vi "FPGA_SuspensionCurrentCheck.vi"() -> ()   [LabVIEW 2014]
uses:
  <vilib>/rvi/Memory/Memory_Emulation/nirvimemoryFastEmulation.vi
  <vilib>/rvi/Memory/Memory_Emulation/nirvimemoryEmulation.vi
  <vilib>/rvi/Emulation/niFpgaEmulationIsFPGAContextNoSignature.vi
  <vilib>/rvi/DataTransferAndStorage/Container/Common/niFpgaContainerGetUniqueNameForEmu.vi
  <vilib>/rvi/Emulation/niFpgaProcessEmulError.vi
  <vilib>/rvi/Emulation/niFpgaSctlEmulationGetInTimedLoop.vi
  <vilib>/rvi/errors/nirviReportUnexpectedCaseInternalError (U32).vi
  <vilib>/rvi/eio/common/nirviEmuTemplateMethod_errors.vi
  <vilib>/rvi/interface/RandomDataEmulation/niFpgaRandomDataHandleErrors.vi
  <vilib>/rvi/Emulation/niFpgaGetClockAttributes.vi
  <vilib>/rvi/Emulation/niFpgaEmulationReportErrorSimple.vi
  <vilib>/rvi/Emulation/niFpgaCriticalErrorInLSC.vi
  <vilib>/rvi/DataTransferAndStorage/Container/XNode/niFpgaContainer.xnode
  <vilib>/eio/EIONode/EIONode.xnode
  <vilib>/rvi/interface/RandomDataEmulation/nirviRandomDataFpgaReadWriteTemplate.vi
panel:
  in  "StepPulseIndex":u32
  in  "SampleSleep us":i32
  in  "SampleNumPerStepIn":i32
  in  "StepInNum":i32
  in  "StepIn?":bool
  in  "SampleNumAfterBack":i32
  out "Monitor":i32
  out "PresCurrent":i16
  out "ZPos":i16
  out "Finished?":bool
  out "Arrived?":bool
  in  "sleep us":u32
  in  "stop":bool
  in  "threshold":sgl
  in  "Offset":i16
  in  "SampleNumAfterApproached":i32
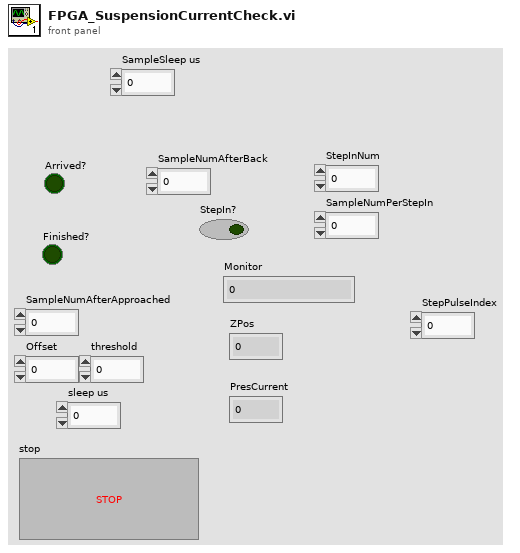
[diagram p1: front panel]
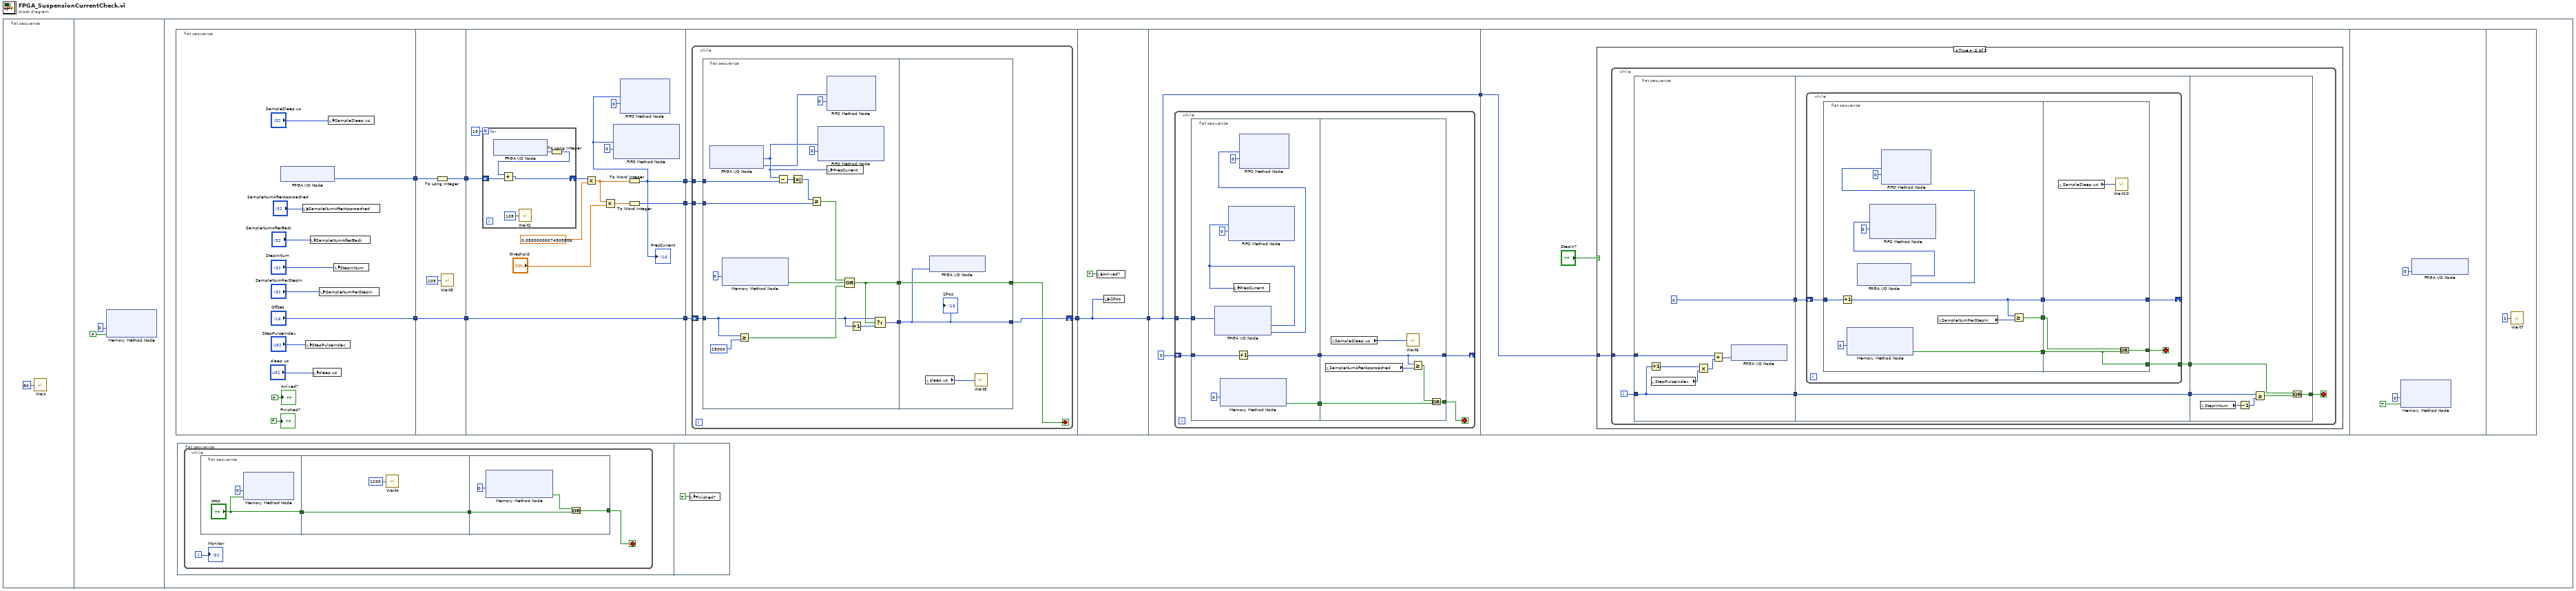
[diagram p0: block diagram]
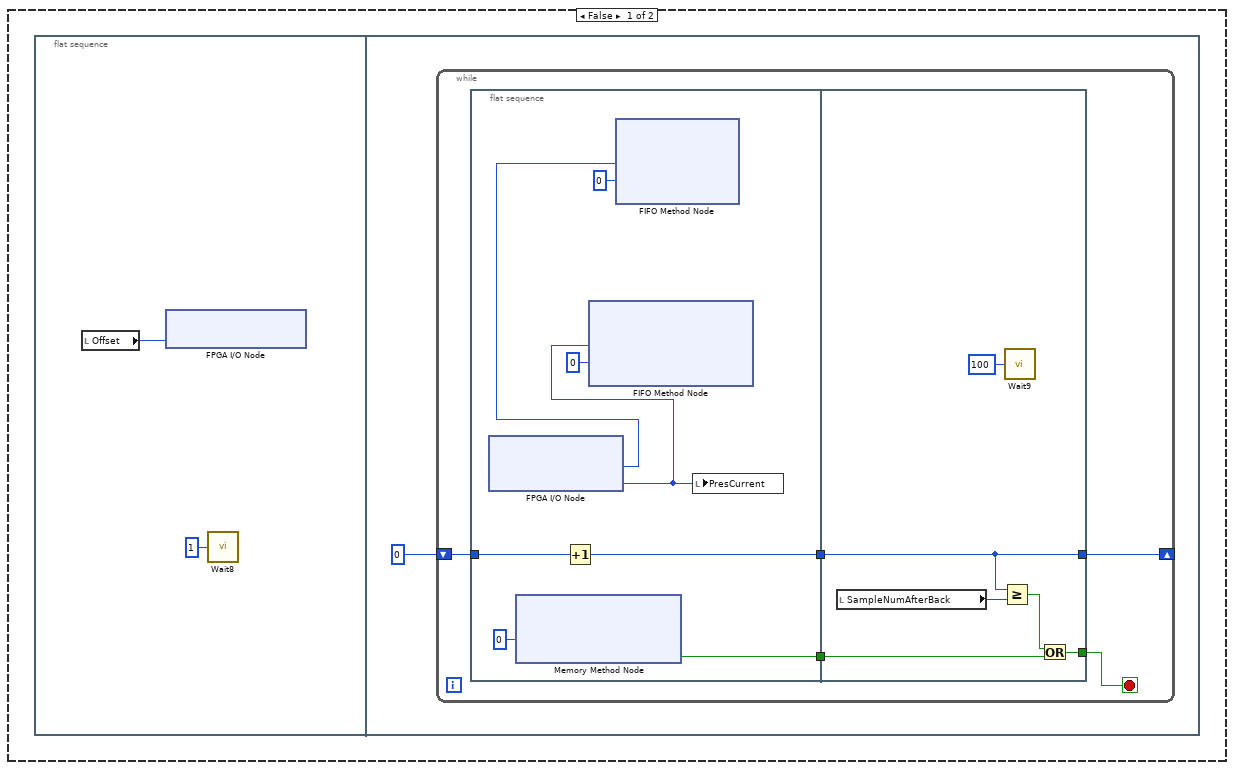
[diagram p2: hidden frame]
diagram:
  n1 = flat-sequence {
    frame #0 {
      n2 = call "Wait"("Count(mSec)"=u32 80) -> ()  [unwired: 1 out]
    }
    frame #1 {
      n3 = xnode ("Memory Method Node")("Address"=u32 0, "Data"=FALSE) -> ()  [unwired: 1 in, 1 out]
    }
    frame #2 {
      n4 = flat-sequence {
        tunnel: ["Offset"] -> w13
        tunnel: [w35] -> w12
        tunnel: w13 -> [w41]
        tunnel: [w41] -> w11
        tunnel: [w38] -> w10
        tunnel: w12 -> [w39]
        tunnel: w11 -> [w53]
        tunnel: [w53] -> w9
        tunnel: w10 -> [w51]
        tunnel: [w43] -> w8
        tunnel: [w45] -> w7
        tunnel: w9 -> [w62]
        tunnel: w8 -> [w61]
        tunnel: w7 -> [w60]
        tunnel: [w59] -> w6
        tunnel: w6 -> [w90]
        tunnel: [w90] -> w5
        tunnel: w5 -> [w92]
        tunnel: [w92] -> w4
        tunnel: w4 -> [w115]
        frame #0 {
          n5 = xnode "FPGA I/O Node"() -> ("Connector0/AI1"=w35:i16)  [unwired: 1 in, 1 out]
          n6 = local write "SampleNumAfterApproached"("SampleNumAfterApproached") -> ()
          n7 = local write "StepPulseIndex"("StepPulseIndex") -> ()
          n8 = local write "SampleNumAfterBack"("SampleNumAfterBack") -> ()
          n9 = local write "sleep us"("sleep us") -> ()
          n10 = local write "SampleNumPerStepIn"("SampleNumPerStepIn") -> ()
          n11 = local write "SampleSleep us"("SampleSleep us") -> ()
          n12 = local write "StepInNum"("StepInNum") -> ()
          "Arrived?" <- FALSE ("Arrived?")
          "Finished?" <- FALSE ("Arrived?")
        }
        frame #1 {
          n13 = To Long Integer(number=w39) -> (32bit integer=w38:i32)
          n14 = call "Wait3"("Count(uSec)"=u32 105) -> ()  [unwired: 1 out]
        }
        frame #2 {
          n15 = for {
            N: 19 -> [_]
            shift-right: [w54] -> w50
            shift-left: w51 -> [w57]
            n16 = xnode "FPGA I/O Node"() -> ("Connector0/AI1"=w56:i16)  [unwired: 1 in, 1 out]
            n17 = call "Wait2"("Count(uSec)"=u32 105) -> ()  [unwired: 1 out]
            n18 = To Long Integer(number=w56) -> (32bit integer=w55:i32)
            n19 = Add(x=w55, y=w57) -> (x+y=w54:i32)
          }
          n20 = Multiply(x=w50, y=sgl 0.05) -> (x*y=w47:sgl)
          n21 = Multiply(x=w47, y="threshold") -> (x*y=w46:sgl)
          n22 = To Word Integer(number=w47) -> (16bit integer=w43:i16)
          "PresCurrent" <- w43
          n23 = xnode ("FIFO Method Node")("Element"=w43, "Timeout"=0) -> ()  [unwired: 1 in, 2 out]
          n24 = xnode ("FIFO Method Node")("Element"=w43, "Timeout"=0) -> ()  [unwired: 1 in, 2 out]
          n25 = To Word Integer(number=w46) -> (16bit integer=w45:i16)
        }
        frame #3 {
          n26 = while {
            shift-right: [w65] -> w59
            shift-left: w62 -> [w67]
            tunnel: w61 -> [w69]
            tunnel: w60 -> [w68]
            stop <- w63 stop-if-true
            n27 = flat-sequence {
              tunnel: w69 -> [w86]
              tunnel: w68 -> [w84]
              tunnel: w67 -> [w76]
              tunnel: [w74] -> w66
              tunnel: [w73] -> w64
              tunnel: w66 -> [w89]
              tunnel: [w89] -> w65
              tunnel: [w87] -> w63
              tunnel: w64 -> [w87]
              frame #0 {
                n28 = xnode "FPGA I/O Node"() -> ("Connector0/AI1"=w72:i16, "Connector0/AI0"=w70:i16)  [unwired: 2 in, 2 out]
                n29 = xnode ("Memory Method Node")("Address"=u32 0) -> ("Data"=w78:bool)  [unwired: 1 in, 1 out]
                n30 = Greater Or Equal?(x=w76, y=i16 29000) -> (x >= y?=w77:bool)
                n31 = Subtract(x=w72, y=w86) -> (x-y=w85:i16)
                n32 = Absolute Value(x=w85) -> (abs(x)=w83:i16)
                n33 = Greater Or Equal?(x=w83, y=w84) -> (x >= y?=w79:bool)
                n34 = xnode ("FIFO Method Node")("Element"=w72, "Timeout"=0) -> ()  [unwired: 1 in, 2 out]
                n35 = xnode ("FIFO Method Node")("Element"=w70, "Timeout"=0) -> ()  [unwired: 1 in, 2 out]
                n36 = local write "PresCurrent"(w72) -> ()
                n37 = Compound Arithmetic op=OR(w79, w78, w77) -> (w73:bool)
                n38 = Increment(x=w76) -> (x+1=w75:i16)
                n39 = Select(t=w76, s=w73, f=w75) -> (s? t:f=w74:i16)
              }
              frame #1 {
                n40 = local read "sleep us"() -> (w88:u32)
                n41 = xnode "FPGA I/O Node"("Connector0/AO0"=w89) -> ()  [unwired: 1 in, 1 out]
                n42 = call "Wait5"("Count(uSec)"=w88) -> ()  [unwired: 1 out]
                "ZPos" <- w89
              }
            }
          }
        }
        frame #4 {
          n43 = local write "Arrived?"(TRUE ("Arrived?")) -> ()
          n44 = local write "ZPos"(w90) -> ()
        }
        frame #5 {
          n45 = while {
            tunnel: w92 -> [w99]
            shift-right: [w94] -> _
            shift-left: 0 -> [w96]
            stop <- w97 stop-if-true
            n46 = flat-sequence {
              tunnel: w99 -> [w108]
              tunnel: [w105] -> w98
              tunnel: w96 -> [w104]
              tunnel: [w103] -> w95
              tunnel: [w112] -> w97
              tunnel: w98 -> [w111]
              tunnel: w95 -> [w113]
              tunnel: [w113] -> w94
              frame #0 {
                n47 = xnode "FPGA I/O Node"("Connector0/AO0"=w108) -> ("Connector0/AI1"=w102:i16, "Connector0/AI0"=w100:i16)  [unwired: 3 in, 3 out]
                n48 = xnode ("Memory Method Node")("Address"=u32 0) -> ("Data"=w105:bool)  [unwired: 1 in, 1 out]
                n49 = xnode ("FIFO Method Node")("Element"=w102, "Timeout"=0) -> ()  [unwired: 1 in, 2 out]
                n50 = local write "PresCurrent"(w102) -> ()
                n51 = Increment(x=w104) -> (x+1=w103:i32)
                n52 = xnode ("FIFO Method Node")("Element"=w100, "Timeout"=0) -> ()  [unwired: 1 in, 2 out]
              }
              frame #1 {
                n53 = local read "SampleNumAfterApproached"() -> (w114:i32)
                n54 = local read "SampleSleep us"() -> (w109:i32)
                n55 = call "Wait6"("Count(uSec)"=w109) -> ()  [unwired: 1 out]
                n56 = Greater Or Equal?(x=w113, y=w114) -> (x >= y?=w110:bool)
                n57 = Or(x=w110, y=w111) -> (x .or. y?=w112:bool)
              }
            }
          }
        }
        frame #6 {
          n58 = case shown="True" "StepIn?" {
            tunnel: w115 -> [_ w139]
            frame False {
              n59 = flat-sequence {
                frame #0 {
                  n60 = local read "Offset"() -> (w118:i16)
                  n61 = xnode "FPGA I/O Node"("Connector0/AO0"=w118) -> ()  [unwired: 1 in, 1 out]
                  n62 = call "Wait8"("Count(mSec)"=u32 1 ("Count(uSec)")) -> ()  [unwired: 1 out]
                }
                frame #1 {
                  n63 = while {
                    shift-right: [w122] -> _
                    shift-left: 0 -> [w124]
                    stop <- w121 stop-if-true
                    n64 = flat-sequence {
                      tunnel: w124 -> [w132]
                      tunnel: [w131] -> w123
                      tunnel: [w129] -> w120
                      tunnel: w123 -> [w138]
                      tunnel: [w138] -> w122
                      tunnel: [w134] -> w121
                      tunnel: w120 -> [w136]
                      frame #0 {
                        n65 = xnode "FPGA I/O Node"() -> ("Connector0/AI0"=w127:i16, "Connector0/AI1"=w128:i16)  [unwired: 2 in, 2 out]
                        n66 = xnode ("Memory Method Node")("Address"=u32 0) -> ("Data"=w129:bool)  [unwired: 1 in, 1 out]
                        n67 = Increment(x=w132) -> (x+1=w131:i32)
                        n68 = xnode ("FIFO Method Node")("Element"=w128, "Timeout"=0) -> ()  [unwired: 1 in, 2 out]
                        n69 = xnode ("FIFO Method Node")("Element"=w127, "Timeout"=0) -> ()  [unwired: 1 in, 2 out]
                        n70 = local write "PresCurrent"(w128) -> ()
                      }
                      frame #1 {
                        n71 = local read "SampleNumAfterBack"() -> (w137:i32)
                        n72 = Greater Or Equal?(x=w138, y=w137) -> (x >= y?=w135:bool)
                        n73 = call "Wait9"("Count(uSec)"=u32 100) -> ()  [unwired: 1 out]
                        n74 = Or(x=w135, y=w136) -> (x .or. y?=w134:bool)
                      }
                    }
                  }
                }
              }
            }
            frame True {
              n75 = while {
                tunnel: w139 -> [w142]
                i -> [w146]
                stop <- w144 stop-if-true
                n76 = flat-sequence {
                  tunnel: w146 -> [w152]
                  tunnel: [w152] -> w143
                  tunnel: w142 -> [w153]
                  tunnel: [i16 0] -> w141
                  tunnel: [w156] -> w145
                  tunnel: w143 -> [w156]
                  tunnel: w141 -> [w155]
                  tunnel: [w154] -> w140
                  tunnel: w145 -> [w184]
                  tunnel: [w179] -> w144
                  tunnel: w140 -> [w180]
                  frame #0 {
                    n77 = Increment(x=w152) -> (x+1=w149:i32)
                    n78 = local read "StepPulseIndex"() -> (w147:u32)
                    n79 = Multiply(x=w149, y=w147) -> (x*y=w148:u32)
                    n80 = Add(x=w153, y=w148) -> (x+y=w151:u32)
                    n81 = xnode "FPGA I/O Node"("Connector0/AO0"=w151) -> ()  [unwired: 1 in, 1 out]
                  }
                  frame #1 {
                    n82 = while {
                      shift-right: [w161] -> _
                      shift-left: w155 -> [w163]
                      tunnel: [w157] -> w154
                      stop <- w158 stop-if-true
                      n83 = flat-sequence {
                        tunnel: w163 -> [w173]
                        tunnel: [w172] -> w162
                        tunnel: [w169] -> w160
                        tunnel: [w168] -> w159
                        tunnel: w162 -> [w178]
                        tunnel: [w178] -> w161
                        tunnel: w160 -> [w174]
                        tunnel: w159 -> [w177]
                        tunnel: [w176] -> w158
                        tunnel: [w174] -> w157
                        frame #0 {
                          n84 = Increment(x=w173) -> (x+1=w172:i16)
                          n85 = xnode ("Memory Method Node")("Address"=u32 0) -> ("Data"=w169:bool)  [unwired: 1 in, 1 out]
                          n86 = xnode "FPGA I/O Node"() -> ("Connector0/AI1"=w167:i16, "Connector0/AI0"=w165:i16)  [unwired: 2 in, 2 out]
                          n87 = xnode ("FIFO Method Node")("Element"=w167, "Timeout"=0) -> ()  [unwired: 1 in, 2 out]
                          n88 = xnode ("FIFO Method Node")("Element"=w165, "Timeout"=0) -> ()  [unwired: 1 in, 2 out]
                          n89 = local read "SampleNumPerStepIn"() -> (w171:i32)
                          n90 = Greater Or Equal?(x=w172, y=w171) -> (x >= y?=w168:bool)
                        }
                        frame #1 {
                          n91 = local read "SampleSleep us"() -> (w175:i32)
                          n92 = call "Wait10"("Count(uSec)"=w175) -> ()  [unwired: 1 out]
                          n93 = Or(x=w177, y=w174) -> (x .or. y?=w176:bool)
                        }
                      }
                    }
                  }
                  frame #2 {
                    n94 = local read "StepInNum"() -> (w182:i32)
                    n95 = Decrement(x=w182) -> (x-1=w183:i32)
                    n96 = Greater Or Equal?(x=w184, y=w183) -> (x >= y?=w181:bool)
                    n97 = Or(x=w180, y=w181) -> (x .or. y?=w179:bool)
                  }
                }
              }
            }
          }
        }
        frame #7 {
          n98 = xnode ("Memory Method Node")("Address"=u32 0, "Data"=TRUE) -> ()  [unwired: 1 in, 1 out]
          n99 = xnode "FPGA I/O Node"("Connector0/AO0"=i16 0) -> ()  [unwired: 1 in, 1 out]
        }
        frame #8 {
          n100 = call "Wait7"("Count(mSec)"=u32 1 ("Count(uSec)")) -> ()  [unwired: 1 out]
        }
      }
      n101 = flat-sequence {
        frame #0 {
          n102 = while {
            i -> [w15]
            stop <- w16 stop-if-true
            n103 = flat-sequence {
              tunnel: ["stop"] -> w17
              tunnel: [w20] -> w14
              tunnel: w17 -> [w20]
              tunnel: [w23] -> w16
              tunnel: w14 -> [w24]
              frame #0 {
                n104 = xnode ("Memory Method Node")("Address"=u32 0, "Data"="stop") -> ()  [unwired: 1 in, 1 out]
              }
              frame #1 {
                n105 = call "Wait4"("Count(uSec)"=u32 1200) -> ()  [unwired: 1 out]
              }
              frame #2 {
                n106 = xnode ("Memory Method Node")("Address"=u32 0) -> ("Data"=w22:bool)  [unwired: 1 in, 1 out]
                n107 = Or(x=w22, y=w24) -> (x .or. y?=w23:bool)
              }
            }
            "Monitor" <- w15
          }
        }
        frame #1 {
          n108 = local write "Finished?"(TRUE ("Finished?")) -> ()
        }
      }
    }
  }
